vi "MB Shutdown.vi"(8 "error in (no error)":errorcluster, 11 "Devices":T1) -> (0 "error out":errorcluster)   [LabVIEW 2021]
uses:
  <vilib>/NI/Modbus Library/API/Master/Modbus Master.lvclass
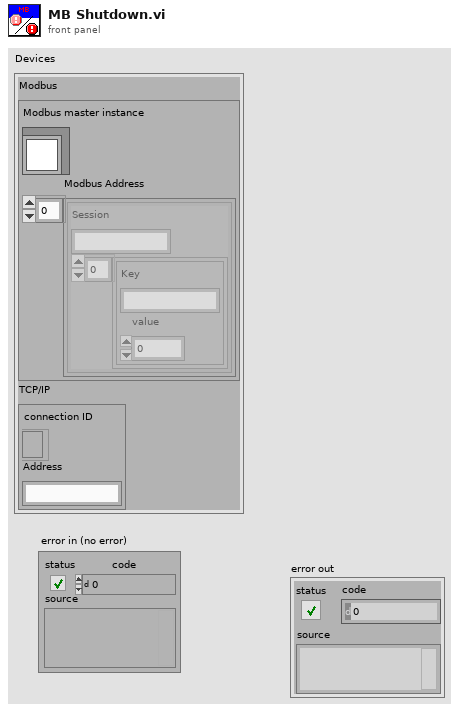
[diagram p1: front panel]
types:
  T1 = cluster{"Modbus":cluster{"Modbus master instance":refnum<class "Modbus Master.lvclass">, "Modbus Address":cluster{"Session":string, cluster{"Key":string, "value":u32}[]}[]}, "TCP/IP":cluster{"connection ID":refnum<k5>, "Address":string}}
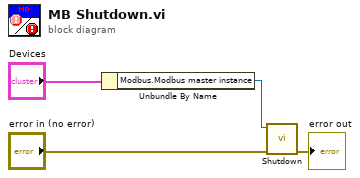
[diagram p0: block diagram]
diagram:
  n1 = Unbundle By Name("Devices") -> ("Modbus.Modbus master instance"=w4:refnum<class "Modbus Master.lvclass">)
  n2 = call-dynamic "Shutdown.vi"("error in"="error in (no error)", "Modbus master in"=w4) -> ("error out"=→"error out":errorcluster)  [unwired: 9 in]
